vi "Initialize.vi"(5 "Password":string, 6 "Force online? (true)":bool=TRUE, 7 "Username (\"\" : target default)":string, 8 "error in (no error)":errorcluster, 11 "Target":refnum<k21>) -> (0 "error out":errorcluster, 2 "Status":string, 3 "RT Management out":refnum<class "RT Management.lvclass">)   [LabVIEW 2015, in "SMI.lvlib"]
doc: "Initializes a connection to the RT target using the System Configuration API. If the username is left blank, then the target defaults are used (even for Linux RT). \"Force online?\" ensures that the system is online and that the RT Management session doesn't continue along using cached System Configuration API properties."
uses:
  SMI.lvlib
  RT Management.lvclass
  <vilib>/nisyscfg/nisyscfg.lvlib
  <resource>/objmgr/nisysapi.rc
  <vilib>/nisyscfg/Close (System).vi
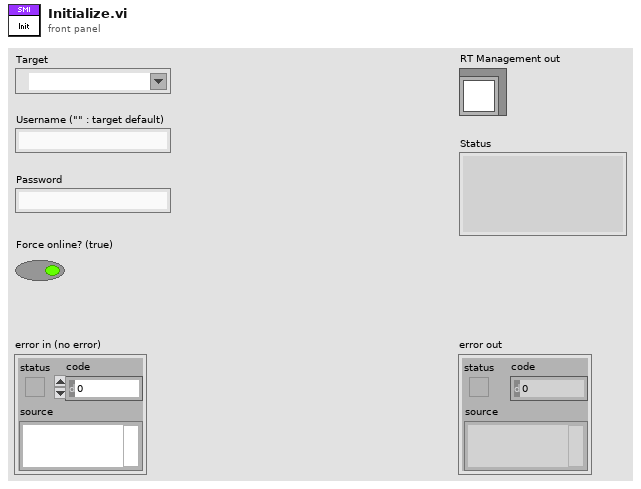
[diagram p1: front panel]
types:
  T1 = typedef "RT Management.lvlib/RT Management.lvclass/Operating system.ctl" = enum16{"Unknown", "VxWorks", "PharLap", "Linux-ARM", "Linux-x64"}
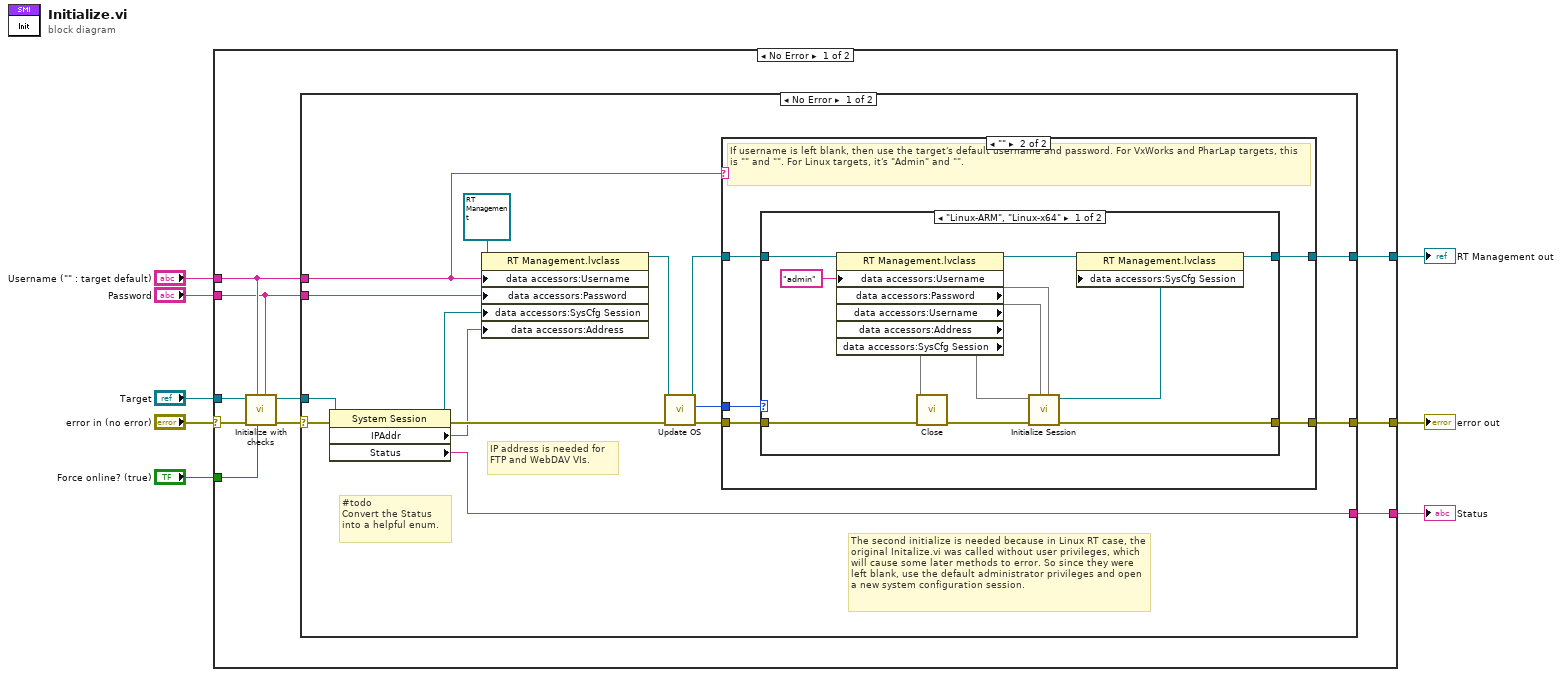
[diagram p0: block diagram]
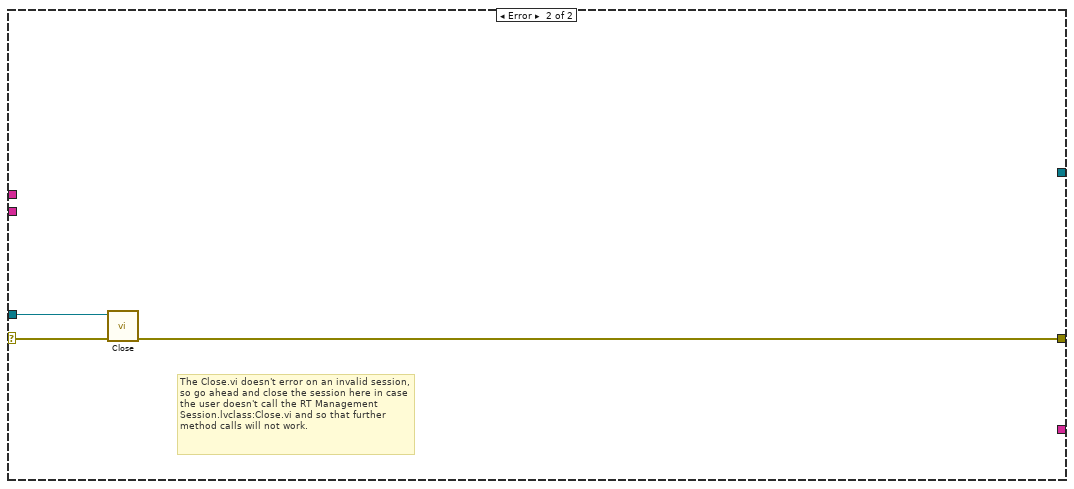
[diagram p4: hidden frame]
diagram:
  n1 = case shown="No Error" "error in (no error)" {
    selector: "error in (no error)" -> [w18 w58]
    tunnel: [w17 w58] -> w7
    tunnel: "Password" -> [w13 _]
    tunnel: "Target" -> [w12 _]
    tunnel: "Username (\"\" : target default)" -> [w14 _]
    tunnel: [w16 _] -> w1
    tunnel: "Force online? (true)" -> [w9 _]
    tunnel: [w15 _] -> w2
    frame No Error {
      n2 = call "Initialize with checks.vi"("Password"=w13, "Force online? (true)"=w9, "Username"=w14, "error in (no error)"=w18, "System Session in"=w12) -> ("error out"=w11:errorcluster, "System Session out"=w10:refnum<k21>)  [unwired: 5 in]
      n3 = case shown="No Error" w11 {
        selector: w11 -> [w23 w55]
        tunnel: [w32 w56] -> w17
        tunnel: [w31 _] -> w16
        tunnel: [w29 _] -> w15
        tunnel: w14 -> [w27 _]
        tunnel: w13 -> [w26 _]
        tunnel: w10 -> [w24 w57]
        frame No Error {
          # "#todo\nConvert the Status into a helpful enum."
          # "The second initialize is needed because in Linux RT case, the original Initalize.vi was called without user privileges, which will cause some later methods to error. So since they were left blank, use the default administrator privileges and open a new system configuration session."
          # "IP address is needed for FTP and WebDAV VIs."
          n4 = property class="System Session"(reference=w24, error in=w23) -> (reference out=w28:refnum<k21>, error out=w33:errorcluster, "IPAddr"=w25:string, "Status"=w29:string)
          n5 = property class="RT Management.lvclass"(reference=refnum<class "RT Management.lvclass"> refnum ("File Transfer Session.lvclass"), "data accessors:Username"=w27, "data accessors:Password"=w26, "data accessors:SysCfg Session"=w28, "data accessors:Address"=w25) -> (reference out=w22:refnum<class "RT Management.lvclass">)  [unwired: 1 in, 1 out]
          n6 = call "Update OS.vi"("error in (no error)"=w33, "RT Management in"=w22) -> ("error out"=w20:errorcluster, "Operating System"=w19:T1, "RT Management out"=w21:refnum<class "RT Management.lvclass">)  [unwired: 6 in, 1 out]
          n7 = case shown="\"\"" w27 {
            tunnel: [w35 w39] -> w32
            tunnel: w20 -> [w35 w37]
            tunnel: w21 -> [w34 w36]
            tunnel: [w34 w40] -> w31
            tunnel: w19 -> [_ w38]
            frame Default {
              # "User provided a non-empty string for the username."
            }
            frame "" {
              # "If username is left blank, then use the target's default username and password. For VxWorks and PharLap targets, this is \"\" and \"\". For Linux targets, it's \"Admin\" and \"\"."
              n8 = case shown="\"Linux-ARM\", \"Linux-x64\"" w38 {
                tunnel: w37 -> [w46 w53]
                tunnel: w36 -> [w42 w54]
                tunnel: [w45 w54] -> w40
                tunnel: [w44 w53] -> w39
                frame "Linux-ARM", "Linux-x64" {
                  n9 = property class="RT Management.lvclass"(reference=w42, "data accessors:Username"="admin" ("username")) -> (reference out=w43:refnum<class "RT Management.lvclass">, "data accessors:Password"=w51, "data accessors:Username"=w50, "data accessors:Address"=w49, "data accessors:SysCfg Session"=w41)  [unwired: 1 in, 1 out]
                  n10 = call-poly <vilib>:"Close.vi"("error in (no error)"=w46, "Session in"=w41) -> ("error out"=w48:errorcluster)  [unwired: 9 in]
                  n11 = call <vilib>:"Initialize Session.vi"("Password"=w51, "User Name"=w50, "error in (no error)"=w48, "Target (localhost)"=w49) -> ("error out"=w44:errorcluster, "Session out"=w52:refnum<k21>)  [unwired: 6 in]
                  n12 = property class="RT Management.lvclass"(reference=w43, "data accessors:SysCfg Session"=w52) -> (reference out=w45:refnum<class "RT Management.lvclass">)  [unwired: 1 in, 1 out]
                }
                frame Default {
                }
              }
            }
          }
        }
        frame Error {
          # "The Close.vi doesn't error on an invalid session, so go ahead and close the session here in case the user doesn't call the RT Management Session.lvclass:Close.vi and so that further method calls will not work."
          n13 = call-poly <vilib>:"Close.vi"("error in (no error)"=w55, "Session in"=w57) -> ("error out"=w56:errorcluster)  [unwired: 9 in]
        }
      }
    }
    frame Error {
    }
  }
  "error out" <- w7
  "RT Management out" <- w1
  "Status" <- w2
